vi "demo_SBOM Generation.vi"(11 "Stop Demo":refnum<user-event>) -> ()   [LabVIEW 2020]
panel:
  # "LabVIEW 2026 Q3 - Automated SBOM Generation\n\nLabVIEW 2026 Q3 build specifications include an option to automatically generate a Software Bill of Materials (SBOM) file using the JKI Security Suite when building an application. SBOM files provide a record of VIPM and NIPM dependencies. Note that this feature requires JKI VI Package Manager and is only supported on Windows at this time."
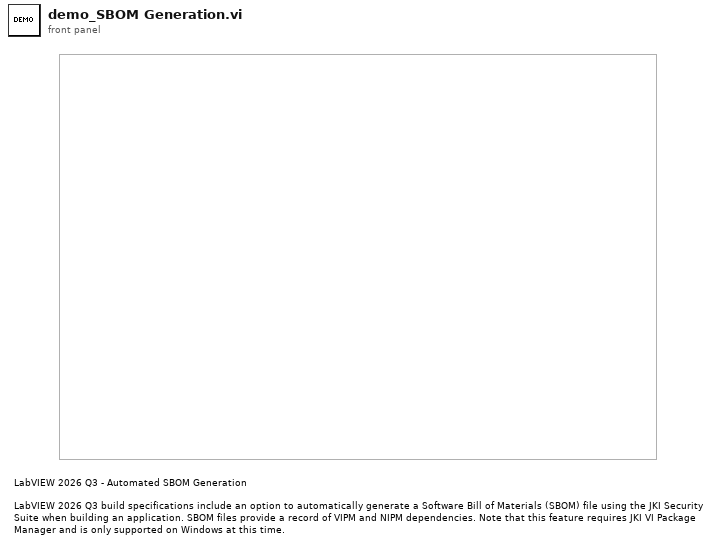
[diagram p1: front panel]
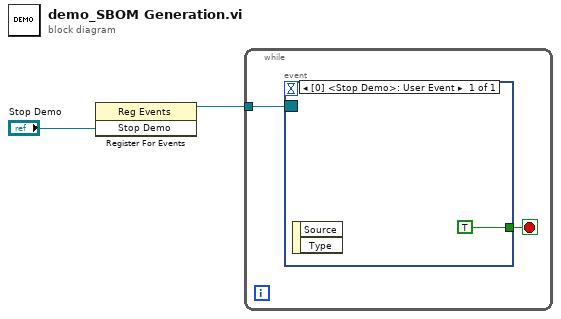
[diagram p0: block diagram]
diagram:
  n1 = register-events("Stop Demo") -> (reference out=w1:refnum<event-registration>)  [unwired: 2 in, 1 out]
  n2 = while {
    tunnel: w1 -> [w4]
    stop <- w3 stop-if-true
    n3 = event shown="[0] <Stop Demo>: User Event" {
      selector: w4 -> [_]
      dyn-events: _ -> [_]
      timeout: _ -> [_]
      tunnel: [TRUE] -> w3
      event User Event {
        n4 = event-data() -> ()  [unwired: 1 in, 2 out]
      }
    }
  }
